vi "Fetch Trace.vi"(8 "error in (no error)":errorcluster, 9 "Timeout (10000 ms)":u32=10000, 11 "VISA resource name":refnum<visa-resource-name>) -> (0 "error out":errorcluster, 2 "Trace Array":sgl[](array[numeric]), 3 "VISA resource name out":refnum<visa-resource-name>, 5 "X Increment":dbl, 7 "Initial X":dbl)   [LabVIEW 2020, in "Template - Spectrum Analyzer.lvlib"]
doc: "Returns the acquired trace and scaling information from the spectrum analyzer. The trace is from an acquisition that you initiate prior to calling this VI. You initiate an acquisition with the <b>Initiate</b> VI.\n\n<B>Note:</B> \n\nUse this VI only with other low-level VIs. The high-level VIs automatically incorporate this functionality. This VI does not check the instrument status."
uses:
  <instrlib>/_Template - Spectrum Analyzer/Template - Spectrum Analyzer.lvlib
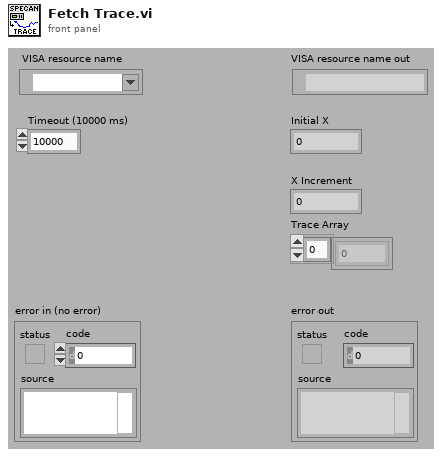
[diagram p1: front panel]
types:
  T1 = enum16{"big-endian, network order", "native, host order", "little-endian"}
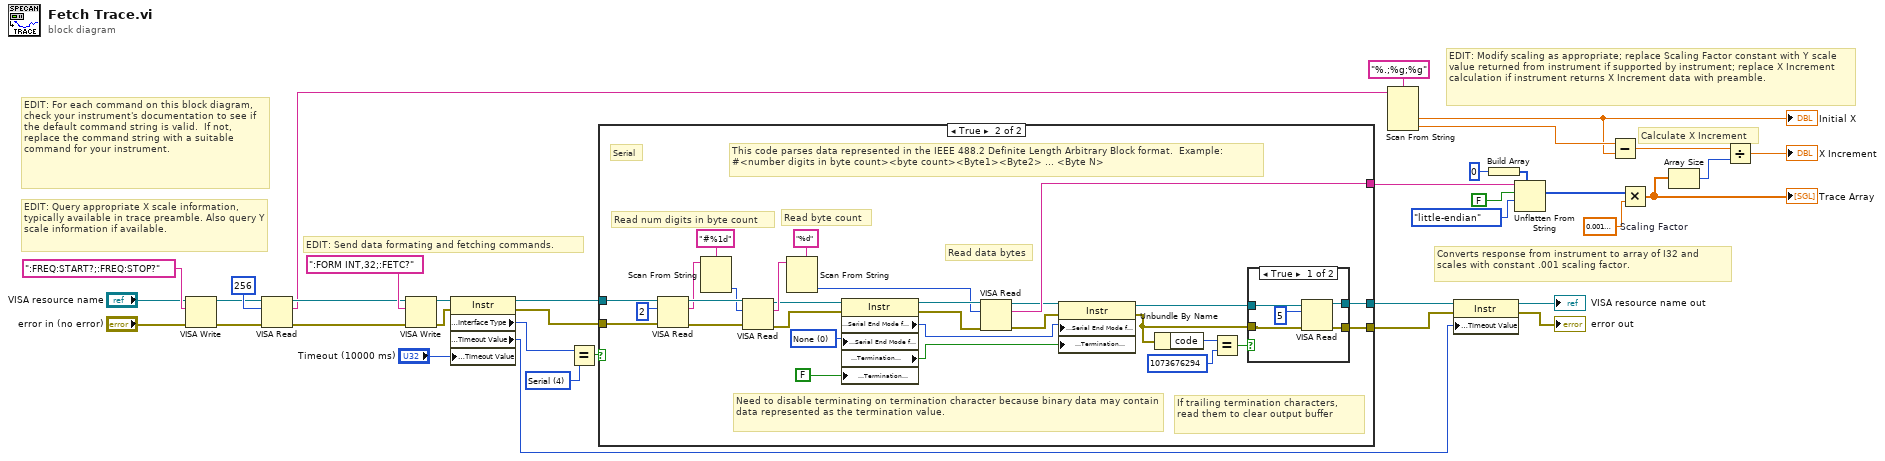
[diagram p0: block diagram]
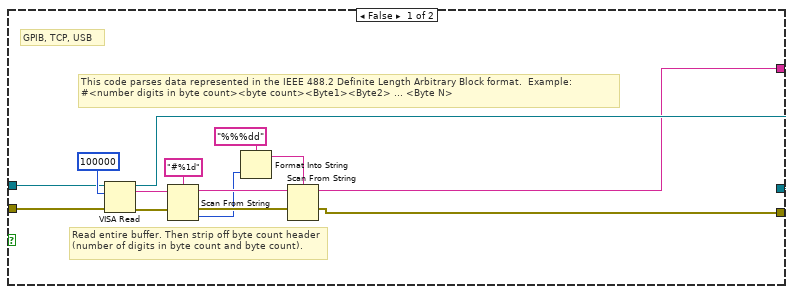
[diagram p2: hidden frame]
diagram:
  w16 = sgl 0.001  # Scaling Factor
  w32 = u16 4 items=["GPIB"=1, "VXI"=2, "GPIB-VXI"=3, "Serial"=4, "PXI"=5, "TCPIP"=6, "USB"=7] ("Interface Information:Interface Type")
  # "EDIT: Query appropriate X scale information, typically available in trace preamble. Also query Y scale information if available."
  # "Converts response from instrument to array of I32 and scales with constant .001 scaling factor."
  # "EDIT: Modify scaling as appropriate; replace Scaling Factor constant with Y scale value returned from instrument if supported by instrument; replace X Increment calculation if instrument returns X Increment data with preamble."
  # "Calculate X Increment"
  # "EDIT: Send data formating and fetching commands."
  # "EDIT: For each command on this block diagram, check your instrument's documentation to see if the default command string is valid.  If not, replace the command string with a suitable command for your instrument."
  n1 = VISA Write(VISA resource name="VISA resource name", write buffer=":FREQ:START?;:FREQ:STOP?", error in (no error)="error in (no error)") -> (VISA resource name out=w12:refnum<visa-resource-name>, error out=w7:errorcluster)  [unwired: 1 out]
  n2 = VISA Read(VISA resource name=w12, byte count=u32 256, error in (no error)=w7) -> (VISA resource name out=w11:refnum<visa-resource-name>, read buffer=w5:string, error out=w10:errorcluster)  [unwired: 1 out]
  n3 = VISA Write(VISA resource name=w11, write buffer=":FORM INT,32;:FETC?" ("Fetch Measurement"), error in (no error)=w10) -> (VISA resource name out=w35:refnum<visa-resource-name>, error out=w34:errorcluster)  [unwired: 1 out]
  n4 = property class="Instr"(reference=w35, error in=w34, "General Settings:Timeout Value"="Timeout (10000 ms)") -> (reference out=w30:refnum<visa-resource-name>, error out=w28:errorcluster, "Interface Information:Interface Type"=w29:u16, "General Settings:Timeout Value"=w22:u32)
  n5 = Equal?(x=w29, y=w32) -> (x = y?=w31:bool)
  n6 = case shown="True" w31 {
    tunnel: w30 -> [w42 w80]
    tunnel: w28 -> [w41 w79]
    tunnel: [w39 w68] -> w19
    tunnel: [w40 w67] -> w21
    tunnel: [w38 w66] -> w23
    frame False {
      # "Read entire buffer. Then strip off byte count header (number of digits in byte count and byte count)."
      # "This code parses data represented in the IEEE 488.2 Definite Length Arbitrary Block format.  Example:  #<number digits in byte count><byte count><Byte1><Byte2> ... <Byte N>"
      # "GPIB, TCP, USB"
      n7 = VISA Read(VISA resource name=w42, byte count=u32 100000, error in (no error)=w41) -> (VISA resource name out=w40:refnum<visa-resource-name>, read buffer=w45:string, error out=w43:errorcluster)  [unwired: 1 out]
      n8 = Scan From String(format string="#%1d", input string=w45, error in=w43) -> (remaining string=w49:string, error out=w47:errorcluster, output 1=w46:i32)  [unwired: 2 in, 1 out]
      n9 = Format Into String(format string="%%%dd", w46) -> (resulting string=w48:string)  [unwired: 2 in, 1 out]
      n10 = Scan From String(format string=w48, input string=w49, error in=w47) -> (remaining string=w38:string, error out=w39:errorcluster)  [unwired: 3 in, 1 out]
    }
    frame True {
      w57 = u16 0 items=["None", "Last Bit", "TermChar"] ("Serial Settings:Serial End Mode for Reads")
      # "Read data bytes"
      # "Read num digits in byte count"
      # "Read byte count"
      # "This code parses data represented in the IEEE 488.2 Definite Length Arbitrary Block format.  Example:  #<number digits in byte count><byte count><Byte1><Byte2> ... <Byte N>"
      # "Need to disable terminating on termination character because binary data may contain data represented as the termination value."
      # "Serial"
      # "If trailing termination characters, read them to clear output buffer"
      n11 = VISA Read(VISA resource name=w80, byte count=u32 2, error in (no error)=w79) -> (VISA resource name out=w75:refnum<visa-resource-name>, read buffer=w65:string, error out=w76:errorcluster)  [unwired: 1 out]
      n12 = Scan From String(format string="#%1d", input string=w65) -> (output 1=w74:i32)  [unwired: 3 in, 3 out]
      n13 = VISA Read(VISA resource name=w75, byte count=w74, error in (no error)=w76) -> (VISA resource name out=w55:refnum<visa-resource-name>, read buffer=w73:string, error out=w54:errorcluster)  [unwired: 1 out]
      n14 = Scan From String(format string="%d", input string=w73) -> (output 1=w56:i32)  [unwired: 3 in, 3 out]
      n15 = property class="Instr"(reference=w55, error in=w54, "Serial Settings:Serial End Mode for Reads"=w57, "Message Based Settings:Termination Character Enable"=FALSE) -> (reference out=w61:refnum<visa-resource-name>, error out=w62:errorcluster, "Serial Settings:Serial End Mode for Reads"=w60:u16, "Message Based Settings:Termination Character Enable"=w53:bool)
      n16 = VISA Read(VISA resource name=w61, byte count=w56, error in (no error)=w62) -> (VISA resource name out=w59:refnum<visa-resource-name>, read buffer=w66:string, error out=w58:errorcluster)  [unwired: 1 out]
      n17 = property class="Instr"(reference=w59, error in=w58, "Serial Settings:Serial End Mode for Reads"=w60, "Message Based Settings:Termination Character Enable"=w53) -> (reference out=w64:refnum<visa-resource-name>, error out=w63:errorcluster)
      n18 = Unbundle By Name(w63) -> ("code"=w71:i32)
      n19 = Equal?(x=w71, y=1073676294 ("code")) -> (x = y?=w69:bool)
      n20 = case shown="True" w69 {
        tunnel: w64 -> [w85 w87]
        tunnel: w63 -> [w81 w86]
        tunnel: [w83 w87] -> w67
        tunnel: [w82 w86] -> w68
        frame True {
          n21 = VISA Read(VISA resource name=w85, byte count=u32 5, error in (no error)=w81) -> (VISA resource name out=w83:refnum<visa-resource-name>, error out=w82:errorcluster)  [unwired: 2 out]
        }
        frame False {
        }
      }
    }
  }
  n22 = Scan From String(format string="%.;%g;%g", input string=w5) -> (output 1=w3:dbl, output 2=w4:dbl)  [unwired: 4 in, 3 out]
  "Initial X" <- w3
  n23 = property class="Instr"(reference=w21, error in=w19, "General Settings:Timeout Value"=w22) -> (reference out=→"VISA resource name out":refnum<visa-resource-name>, error out=→"error out":errorcluster)
  n24 = Build Array(0) -> (w24:i32[])
  n25 = Unflatten From String(type=w24, binary string=w23, data includes array or string size? (T)=FALSE, byte order (0:big-endian, network order)=T1."little-endian") -> (value=w17:i32[])  [unwired: 1 in, 2 out]
  n26 = Subtract(x=w4, y=w3) -> (x-y=w15:dbl)
  n27 = Multiply(x=w17, y=w16) -> (x*y=w2:sgl[])
  "Trace Array" <- w2
  n28 = Array Size(array=w2) -> (size(s)=w14:i32)
  n29 = Divide(x=w15, y=w14) -> (x/y=→"X Increment":dbl)
